vi "rszvl Query ViString.vi"(8 "error in (no error)":errorcluster, 10 "Command":string, 11 "VISA resource name":refnum<visa-resource-name>) -> (0 "error out":errorcluster, 2 "Value":string, 3 "VISA resource name out":refnum<visa-resource-name>)   [LabVIEW 2014]
doc: "This VI sends the SCPI query to the instrument, and reads the response. The response is trimmed of leading and trailing white characters (\\n, \\r, \\t, \\s).\nThe length of the response is not limited. If it is longer than 65kB, the transfer is performed over VISA interface in 65kB bytes long chunks and combined together.\nDo not use this VI if you expect binary data response (data starting with # character) e.g. file data content or trace data. For that purpose use <b>Read To File From Instrument.vi</b> or more general <b>Bin Data To File From Instrument.vi</b>"
uses:
  rszvl_rsidr_core.lvlib
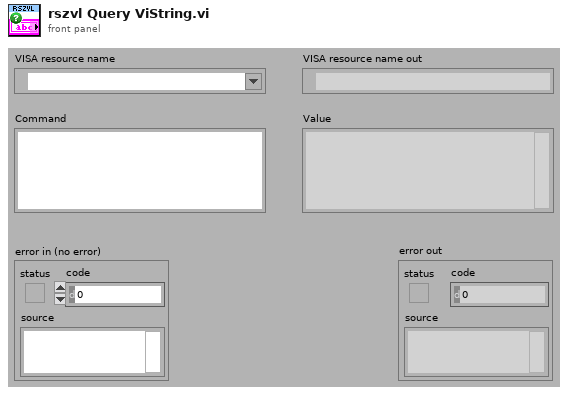
[diagram p1: front panel]
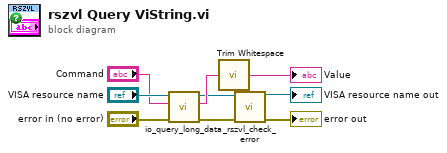
[diagram p0: block diagram]
diagram:
  n1 = call "io_query_long_data.vi"("error in"="error in (no error)", "write buffer"="Command", "VISA resource name"="VISA resource name") -> ("error out"=w7:errorcluster, "read buffer"=w5:string, "VISA resource name out"=w3:refnum<visa-resource-name>)  [unwired: 6 in]
  n2 = call "Trim Whitespace.vi"("string"=w5) -> ("trimmed string"=→"Value":string)  [unwired: 1 in]
  n3 = call "_rszvl_check_error.vi"("VISA resource name"=w3, "error in"=w7) -> ("VISA resource name out"=→"VISA resource name out":refnum<visa-resource-name>, "error out"=→"error out":errorcluster)  [unwired: 12 in]
